vi "AVS_Read_Resistance.vi"(4 "AVS-Excitation":i8, 6 "error in (no error)":errorcluster caption="Fehler (Eingang, kein Fehler)", 7 "Wait for channel (s)":i8, 8 "AVS Channel":i8, 9 "AVS-VISA":refnum<visa-resource-name>) -> (0 "error out":errorcluster caption="Fehler (Ausgang)", 2 "AVS Resistance reading":dbl format="%.2f", 3 "dup AVS-VISA":refnum<visa-resource-name>)   [LabVIEW 2018]
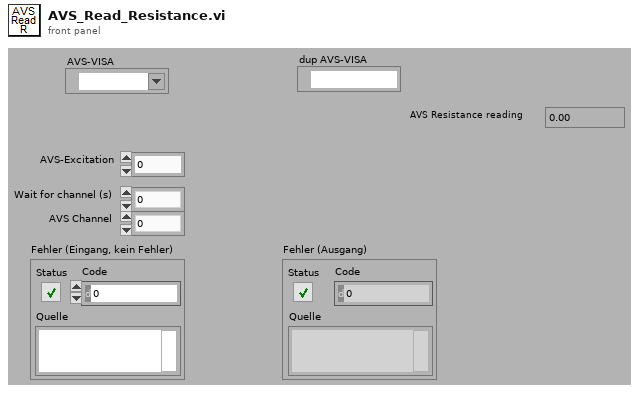
[diagram p1: front panel]
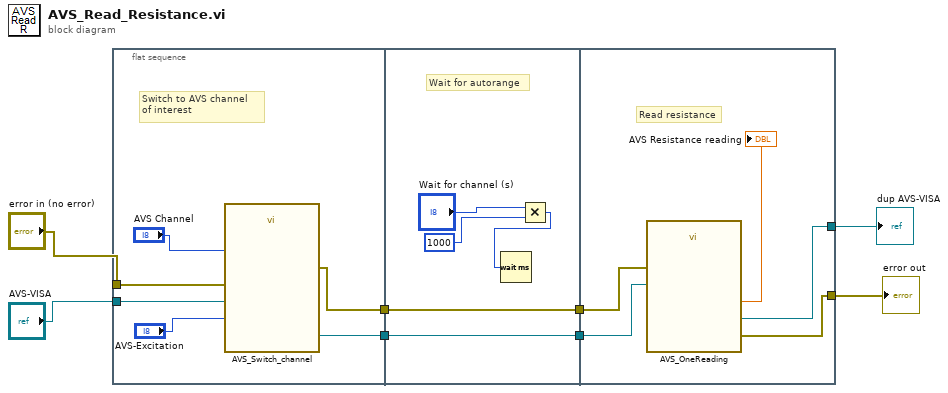
[diagram p0: block diagram]
diagram:
  n1 = flat-sequence {
    tunnel: [w13] -> w7
    tunnel: "error in (no error)" -> [w12]
    tunnel: "AVS-VISA" -> [w11]
    tunnel: [w9] -> w2
    tunnel: [w16] -> w8
    tunnel: w7 -> [w16]
    tunnel: [w15] -> w3
    tunnel: w2 -> [w15]
    tunnel: w8 -> [w23]
    tunnel: [w20] -> w6
    tunnel: w3 -> [w24]
    tunnel: [w21] -> w1
    frame #0 {
      # "Switch to AVS channel \nof interest"
      n2 = call "AVS_Switch_channel.vi"("error in (no error) 3"=w12, "AVS Excitation"="AVS-Excitation", "AVS Channel"="AVS Channel", "AVS-VISA"=w11) -> ("error out (no error) 2"=w13:errorcluster, "dup VISA-AVS"=w9:refnum<visa-resource-name>)  [unwired: 6 in]
    }
    frame #1 {
      # "Wait for autorange"
      n3 = Multiply(x="Wait for channel (s)", y=1000) -> (x*y=w17:i32)
      n4 = Wait (ms)(milliseconds to wait=w17) -> ()  [unwired: 1 out]
    }
    frame #2 {
      # "Read resistance"
      n5 = call "AVS_OneReading.vi"("error in (no error) 4"=w23, "AVS-VISA"=w24) -> ("error out (no error)"=w20:errorcluster, "AVS Resistance reading"=→"AVS Resistance reading":dbl, "dup AVS-VISA"=w21:refnum<visa-resource-name>)  [unwired: 3 in]
    }
  }
  "error out" <- w6
  "dup AVS-VISA" <- w1
